vi "Preview Build.vi"(8 "error in (no error)":errorcluster, 11 "Build Package Step in":refnum<class "Build Package Step.lvclass">) -> (0 "error out":errorcluster, 2 "Artifacts":refnum<class "Build Artifact.lvclass">[](array[class]))   [LabVIEW 2019, in "VIPM.lvlib" / "Build Package Step.lvclass"]
doc: "Gets a preview of the build. This should return as much information about the artifacts as possible without actually building.\n\nDo not perform any actions that may take a long amount of time.\n\nCopyright: MGI 2016\nAuthor: Derek Trepanier"
uses:
  Build Package Step.lvclass
  libs/Solution.lvlibp/Solution/Build Artifact/Build Artifact.lvclass
  <vilib>/xml/NI_XML.lvlib
  <vilib>/xml/Load XML File.vi
  <vilib>/xml/Close Reference(Node).vi
  libs/Project.lvlibp/Project/Binary File/Binary File.lvclass
  C:/Users/pasca/source/repos/mgi-solution-explorer-extensions/libs/Solution.lvlibp/Solution/Build Artifact/Build Artifact.lvclass
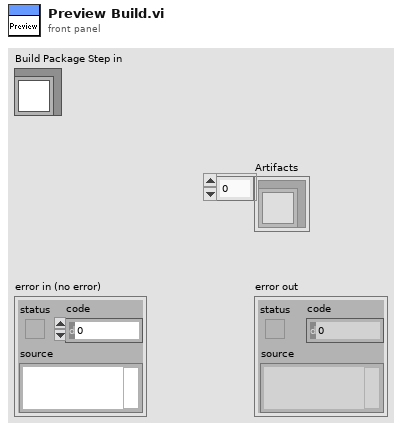
[diagram p1: front panel]
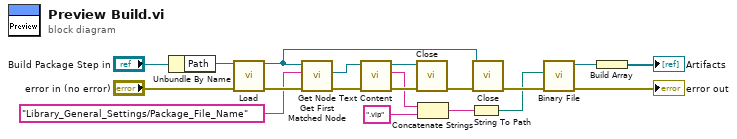
[diagram p0: block diagram]
diagram:
  n1 = Unbundle By Name("Build Package Step in") -> ("Path"=w17:path)
  n2 = call-poly <vilib>:"Load.vi"("path to XML document"=w17, "error in (no error)"="error in (no error)") -> ("DOM document out"=w9:refnum<k20>, "error out"=w16:errorcluster)  [unwired: 11 in, 1 out]
  n3 = call <vilib>:"Get First Matched Node.vi"("error in (no error)"=w16, "XPath expression"="Library_General_Settings/Package_File_Name", "node in"=w9) -> ("error out"=w15:errorcluster, "node result"=w12:refnum<k20>)  [unwired: 6 in, 1 out]
  n4 = call <vilib>:"Get Node Text Content.vi"("error in (no error)"=w15, "node in"=w12) -> ("error out"=w13:errorcluster, "node text"=w4:string, "node out"=w10:refnum<k20>)  [unwired: 7 in]
  n5 = call-poly <vilib>:"Close.vi"("error in (no error)"=w13, "node"=w10) -> ("error out"=w11:errorcluster)  [unwired: 7 in]
  n6 = Concatenate Strings(w4, ".vip" ("string")) -> (w2:string)
  n7 = String To Path(string=w2) -> (path=w1:path)
  n8 = call-poly <vilib>:"Close.vi"("error in (no error)"=w11, "node"=w9) -> ("error out"=w8:errorcluster)  [unwired: 7 in]
  n9 = call "Binary File.vi"("error in (no error)"=w8, "File"=w1) -> ("error out"=→"error out":errorcluster, "Binary File out"=w6:refnum<class "Binary File.lvclass">)  [unwired: 8 in]
  n10 = Build Array(w6) -> (→"Artifacts":refnum<class "Binary File.lvclass">[])
